vi "Get Firmware Version.vi"(8 "Error In":errorcluster, 11 "LINX Device Config":T2) -> (0 "Error Out":errorcluster, 2 "LINX Firmware Version":T1, 3 "LINX Device Config":T2)   [LabVIEW 2014, in "LMH-LINX.lvlib" / "Device.lvlib"]
uses:
  <vilib>/MakerHub/LINX/Private/Device/Device.lvlib
  <vilib>/MakerHub/LINX/Private/Device/Type Defs/LINX Device Config.ctl
  <vilib>/MakerHub/LINX/Private/Type Defs/Interface.ctl
  <vilib>/MakerHub/LINX/Private/Device/Type Defs/TCP Config.ctl
  <vilib>/MakerHub/LINX/Private/Device/Type Defs/Channels.ctl
  <vilib>/MakerHub/LINX/Private/Device/Type Defs/Firmware Version.ctl
  <vilib>/MakerHub/LINX/Private/Type Defs/Error Type.ctl
  <vilib>/MakerHub/LINX/LMH-LINX.lvlib
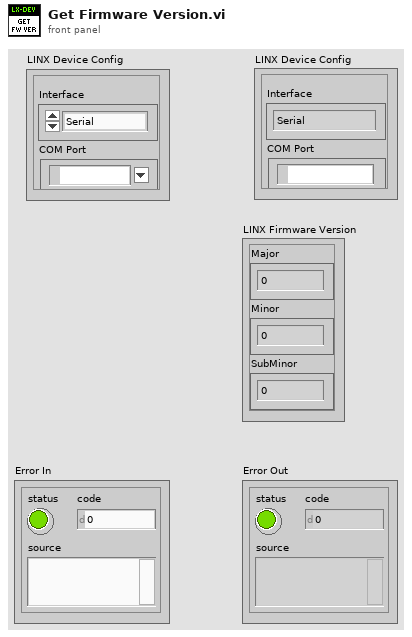
[diagram p1: front panel]
types:
  T1 = typedef "LMH-LINX.lvlib/Device.lvlib/Firmware Version.ctl" = cluster{"Major":u8, "Minor":u8, "SubMinor":u8}
  T2 = typedef "LMH-LINX.lvlib/Device.lvlib/LINX Device Config.ctl" = cluster{"Interface":T3, "COM Port":refnum<visa-resource-name>, "TCP Configuration":T4, "Device Family":u8, "Device ID":u8, "Device Name":string, "TCP Ref":refnum<k5>, "Channels":T5}
  T3 = typedef "LMH-LINX.lvlib/Interface.ctl" = enum16{"Serial", "TCP"}
  T4 = typedef "LMH-LINX.lvlib/Device.lvlib/TCP Config.ctl" = cluster{"IP Address":string, "Port":u16}
  T5 = typedef "LMH-LINX.lvlib/Channels.ctl" = cluster{"DI":u8[], "DO":u8[], "AI":u8[], "AO":u8[], "PWM":u8[], "QE":u8[], "UART":u8[], "I2C 2":u8[], "SPI":u8[], "CAN":u8[], "Servo":u8[], "AI Ref (V)":dbl, "AI Resolution (Bits)":u8, "AO Ref (V)":dbl, "AO Resolution (Bits)":u8}
  T6 = typedef "LMH-LINX.lvlib/Error Type.ctl" = enum16{"Unknown", "Timeout", "Corrupt Return Packet", "Unable To Connect", "Command Not Supported", "Channel DNE", "Invalid COM Config", "Firmware Version Mismatch", "myRIO Support", "CMD Specific Error", "Local IO Not Supported"}
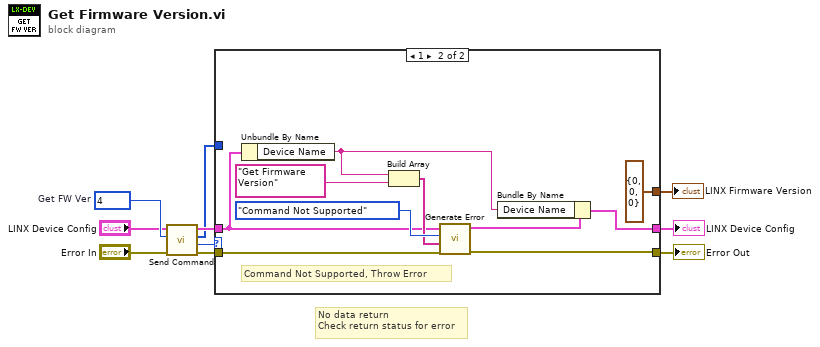
[diagram p0: block diagram]
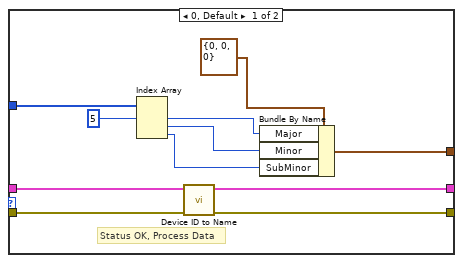
[diagram p2: hidden frame]
diagram:
  w9 = u16 4  # Get FW Ver
  # "No data return\nCheck return status for error"
  n1 = call <vilib>:"Send Command.vi"("Error In"="Error In", "CMD"=w9, "LINX Device Config"="LINX Device Config") -> ("Error Out"=w4:errorcluster, "Status"=w2:u8, "Response"=w3:u8[], "LINX Device Config"=w6:T2)  [unwired: 5 in]
  n2 = case shown="1" w2 {
    tunnel: [w18 w25] -> w7
    tunnel: w6 -> [w21 w24]
    tunnel: [w19 w30] -> w5
    tunnel: w4 -> [w20 w31]
    tunnel: w3 -> [w17 _]
    tunnel: [w11 T1 {"Major"=0, "Minor"=0, "SubMinor"=0} ("LINX Firmware Version")] -> w1
    frame 0, Default {
      # "Status OK, Process Data"
      n3 = Index Array(array=w17, index #1=5 ("index")) -> (element #1=w14:u8, element #2=w13:u8, element #3=w12:u8)  [unwired: 2 in]
      n4 = call <vilib>:"Device ID to Name.vi"("Error In"=w20, "LINX Device Config"=w21) -> ("Error Out"=w19:errorcluster, "LINX Device Config"=w18:T2)  [unwired: 7 in, 1 out]
      n5 = Bundle By Name(cluster=T1 {"Major"=0, "Minor"=0, "SubMinor"=0} ("LINX Firmware Version"), "Major"=w14, "Minor"=w13, "SubMinor"=w12) -> (w11:T1)
    }
    frame 1 {
      # "Command Not Supported, Throw Error"
      n6 = Unbundle By Name(w24) -> ("Device Name"=w23:string)
      n7 = Build Array(w23, "Get Firmware Version") -> (w27:string[])
      n8 = call <vilib>:"Generate Error.vi"("Error In"=w31, "Arguments"=w27, "Error Type"=Error_Type."Command Not Supported", "LINX Device Config"=w24) -> ("Error Out"=w30:errorcluster, "Dup LINX Device Config"=w26:T2)  [unwired: 6 in]
      n9 = Bundle By Name(cluster=w26, "Device Name"=w23) -> (w25:T2)
    }
  }
  "Error Out" <- w5
  "LINX Device Config" <- w7
  "LINX Firmware Version" <- w1
